vi "DAQ AO.vi"(8 "error in":errorcluster, 9 "Config":cluster{"min value":dbl, "max value":dbl}={"min value"=-5.0, "max value"=5.0} {"max value" format="%#_13g"; "min value" format="%#_13g"}, 10 "AO":dbl[](array[numeric]) format="%#_13g", 11 "Alias":string) -> (0 "error out":errorcluster)   [LabVIEW 2021]
uses:
  Controls/DAQ_Data.ctl
  Controls/Measure Type.ctl
  <vilib>/DAQmx/write.llb/DAQmx Write (Analog 1D DBL 1Chan NSamp).vi
  <vilib>/DAQmx/create/channels.llb/DAQmx Create Channel (AO-Voltage-Basic).vi
  <vilib>/DAQmx/miscellaneous.llb/DAQmx Fill In Error Info.vi
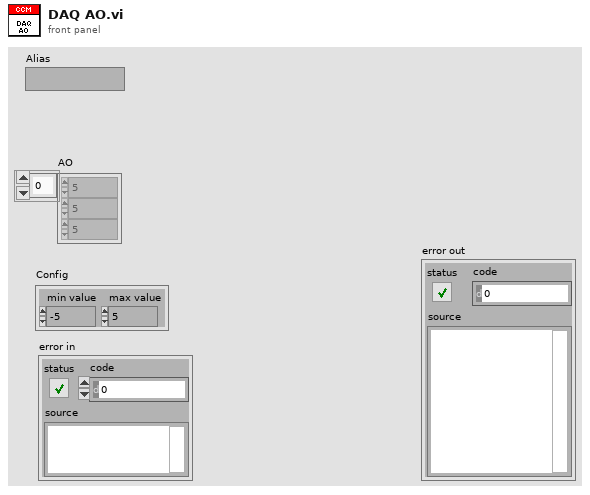
[diagram p1: front panel]
types:
  T1 = typedef "Measure Type.ctl" = enum16{"Analog_In", "Analog_Out", "Digital_In", "Digital_Out", "Switch", "NI_DMM"}
  T2 = typedef "DAQ_Data.ctl" = cluster{"Alias":string, "DAQ Ch":string}
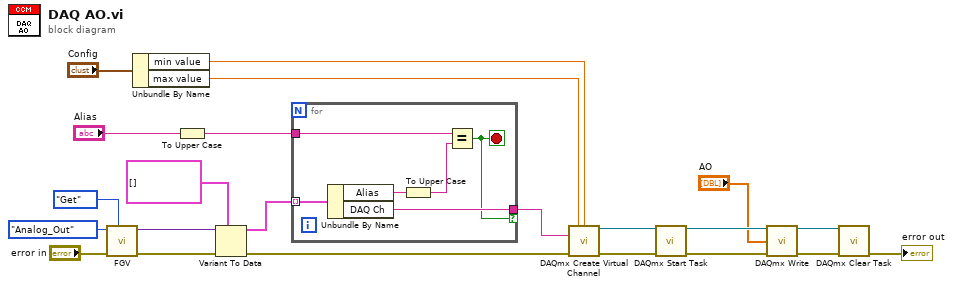
[diagram p0: block diagram]
diagram:
  n1 = call "FGV.vi"("Method (Get)"=enum16{"Get", "Set"}."Get", "error in"="error in", "Name"=Measure_Type."Analog_Out") -> ("error out"=w10:errorcluster, "Data out"=w9:variant)  [unwired: 7 in]
  n2 = Unbundle By Name("Config") -> ("min value"=w16:dbl, "max value"=w15:dbl)
  n3 = To Upper Case(1:"Alias") -> (0:w1:string)
  n4 = Variant To Data(error in=w10, type=T2[] [], Variant=w9) -> (data=w5:T2[], error out=w6:errorcluster)
  n5 = for {
    tunnel: w5 -> [w28] mode=indexing
    tunnel: [w27] -> w3 if=w24
    tunnel: w1 -> [w26]
    stop <- w24 stop-if-true
    n6 = Unbundle By Name(w28) -> ("Alias"=w25:string, "DAQ Ch"=w27:string)
    n7 = To Upper Case(1:w25) -> (0:w23:string)
    n8 = Equal?(x=w26, y=w23) -> (x = y?=w24:bool)
  }
  n9 = call-poly <vilib>:"DAQmx Create Virtual Channel.vi"("maximum value"=w15, "minimum value"=w16, "physical channels"=w3, "error in"=w6) -> ("task out"=w17:refnum<k21>, "error out"=w18:errorcluster)  [unwired: 10 in]
  n10 = call <vilib>:"DAQmx Start Task.vi"("task/channels in"=w17, "error in"=w18) -> ("task out"=w20:refnum<k21>, "error out"=w19:errorcluster)  [unwired: 12 in]
  n11 = call-poly <vilib>:"DAQmx Write.vi"("task/channels in"=w20, "data"="AO", "error in"=w19) -> ("task out"=w14:refnum<k21>, "error out"=w13:errorcluster)  [unwired: 10 in, 1 out]
  n12 = call <vilib>:"DAQmx Clear Task.vi"("task in"=w14, "error in"=w13) -> ("error out"=→"error out":errorcluster)  [unwired: 13 in]
